vi "Routine Before BIST I.vi"(4 "ID Response":string="18DAF255", 5 "ID Request":string="18DA55F2", 6 "Read":refnum<k21>, 7 "Write":refnum<k21>) -> (0 "Data String 3":string, 1 "ID String 3":string, 2 "Write out":refnum<k21>, 3 "Read out":refnum<k21>)   [LabVIEW 2023]
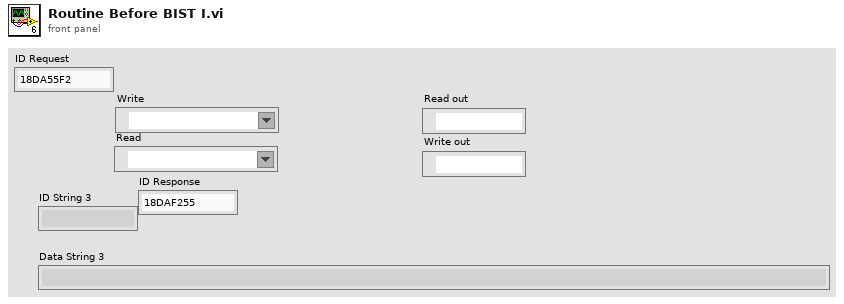
[diagram p1: front panel]
types:
  T1 = typedef "XNET Frame CAN.ctl" = cluster{"timestamp":timestamp, "payload":u8[], "identifier":u32, "type":T2, "extended?":bool, "echo?":bool}
  T2 = typedef "XNET Frame Type CAN.ctl" = u8
  T3 = cluster{"data[0]":T1, "data[1]":T1, "data[2]":T1, "data[3]":T1, "data[4]":T1, "data[5]":T1, "data[6]":T1, "data[7]":T1, "data[8]":T1}
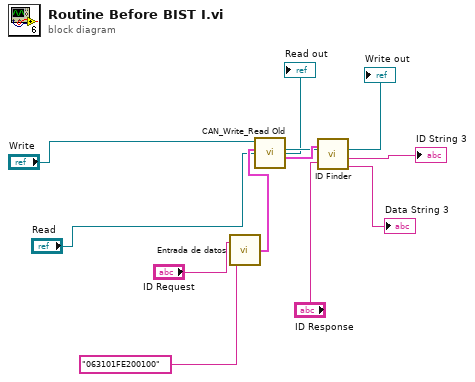
[diagram p0: block diagram]
diagram:
  n1 = call "Entrada de datos.vi"("string"="063101FE200100" ("string 3"), "ID"="ID Request") -> ("CAN frame"=w8:T1)
  n2 = call "CAN_Write_Read Old.vi"("Read In"="Read", "CAN frame"=w8, "Write In"="Write") -> ("cluster"=w9:T3, "Write Out"=→"Write out":refnum<k21>, "Read Out"=→"Read out":refnum<k21>)  [unwired: 2 in, 2 out]
  n3 = call "ID Finder.vi"("cluster"=w9, "ID ESPERADO STRING"="ID Response") -> ("ID String"=→"ID String 3":string, "Data String"=→"Data String 3":string)  [unwired: 4 out]
